vi "move_1ax_thor_z825b.vi"() -> ()   [LabVIEW 2013]
panel:
  in  "fAbsPosCh2":sgl
  out "GetPosition":i32
  out "pfPosition":sgl
  out "error out":errorcluster
  in  "serial":i32
  in  "MG17Motor":refnum<k7>(container)
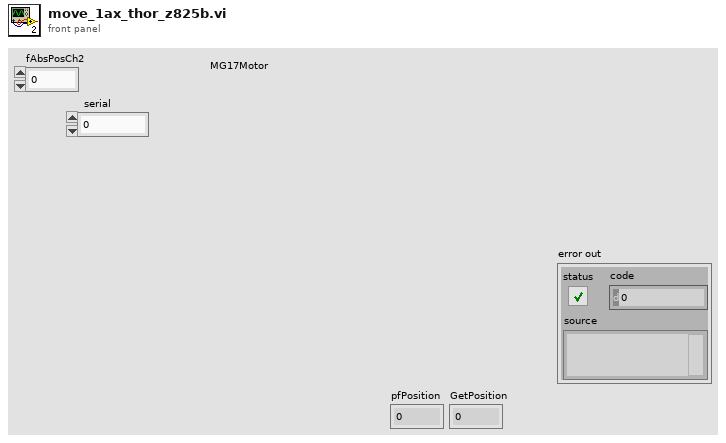
[diagram p1: front panel]
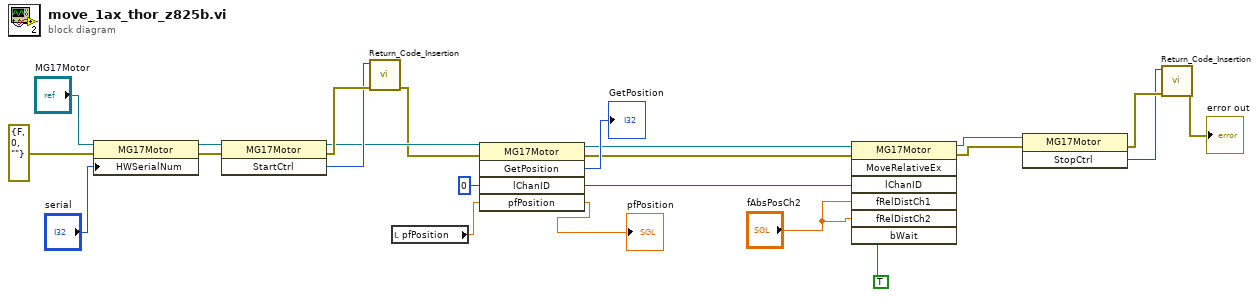
[diagram p0: block diagram]
diagram:
  n1 = property class="MG17Motor"(reference="MG17Motor", error in=errorcluster {"status"=FALSE, "code"=0, "source"=""} ("error in (no error)"), "HWSerialNum"="serial") -> (reference out=w21:refnum<k7>, error out=w19:errorcluster)
  n2 = invoke class="MG17Motor" method="StartCtrl"(reference=w21, error in=w19) -> (reference out=w10:refnum<k7>, error out=w18:errorcluster, "StartCtrl"=w17:i32)  [unwired: 1 in]
  n3 = call "Return_Code_Insertion.vi"("error in (no error)"=w18, "Return Code"=w17) -> ("error out"=w9:errorcluster)  [unwired: 9 in]
  n4 = local read "pfPosition"() -> (w6:sgl)
  n5 = invoke class="MG17Motor" method="GetPosition"(reference=w10, error in=w9, "lChanID"=0, "pfPosition"=w6) -> (reference out=w4:refnum<k7>, error out=w3:errorcluster, "GetPosition"=→"GetPosition":i32, "lChanID"=w7:i32, "pfPosition"=→"pfPosition":sgl)  [unwired: 1 in]
  n6 = invoke class="MG17Motor" method="MoveRelativeEx"(reference=w4, error in=w3, "lChanID"=w7, "fRelDistCh1"="fAbsPosCh2", "fRelDistCh2"="fAbsPosCh2", "bWait"=TRUE) -> (reference out=w13:refnum<k7>, error out=w12:errorcluster)  [unwired: 1 in, 5 out]
  n7 = invoke class="MG17Motor" method="StopCtrl"(reference=w13, error in=w12) -> (error out=w16:errorcluster, "StopCtrl"=w15:i32)  [unwired: 1 in, 1 out]
  n8 = call "Return_Code_Insertion.vi"("error in (no error)"=w16, "Return Code"=w15) -> ("error out"=→"error out":errorcluster)  [unwired: 9 in]
